vi "DriveLoop.vi"   [LabVIEW 2017]
uses:
  <userlib>/836-Library/System/QCP_V2/QCPSupportCode/QCP_GetDblArr.vi
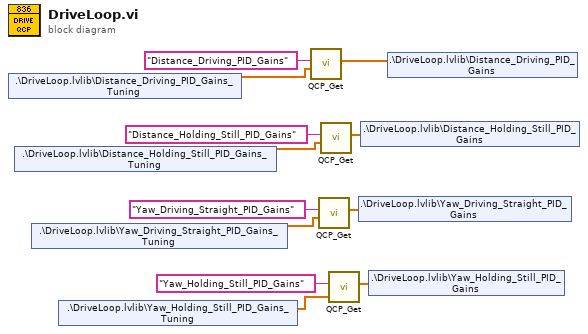
[diagram p0: block diagram]
diagram:
  n1 = shared-variable ".\\DriveLoop.lvlib\\Distance_Driving_PID_Gains_Tuning"() -> (w4:dbl[])  [unwired: 1 in, 1 out]
  n2 = shared-variable ".\\DriveLoop.lvlib\\Distance_Holding_Still_PID_Gains_Tuning"() -> (w3:dbl[])  [unwired: 1 in, 1 out]
  n3 = shared-variable ".\\DriveLoop.lvlib\\Yaw_Driving_Straight_PID_Gains_Tuning"() -> (w2:dbl[])  [unwired: 1 in, 1 out]
  n4 = shared-variable ".\\DriveLoop.lvlib\\Yaw_Holding_Still_PID_Gains_Tuning"() -> (w1:dbl[])  [unwired: 1 in, 1 out]
  n5 = call-poly <userlib>:"QCP_Get.vi"("Tuning Value"=w4, "Value Name"="Distance_Driving_PID_Gains") -> ("Values"=w8:dbl[])  [unwired: 7 in, 2 out]
  n6 = call-poly <userlib>:"QCP_Get.vi"("Tuning Value"=w2, "Value Name"="Yaw_Driving_Straight_PID_Gains") -> ("Values"=w6:dbl[])  [unwired: 7 in, 2 out]
  n7 = call-poly <userlib>:"QCP_Get.vi"("Tuning Value"=w3, "Value Name"="Distance_Holding_Still_PID_Gains") -> ("Values"=w7:dbl[])  [unwired: 7 in, 2 out]
  n8 = call-poly <userlib>:"QCP_Get.vi"("Tuning Value"=w1, "Value Name"="Yaw_Holding_Still_PID_Gains") -> ("Values"=w5:dbl[])  [unwired: 7 in, 2 out]
  n9 = shared-variable ".\\DriveLoop.lvlib\\Yaw_Driving_Straight_PID_Gains"(w6) -> ()  [unwired: 1 in, 1 out]
  n10 = shared-variable ".\\DriveLoop.lvlib\\Distance_Holding_Still_PID_Gains"(w7) -> ()  [unwired: 1 in, 1 out]
  n11 = shared-variable ".\\DriveLoop.lvlib\\Yaw_Holding_Still_PID_Gains"(w5) -> ()  [unwired: 1 in, 1 out]
  n12 = shared-variable ".\\DriveLoop.lvlib\\Distance_Driving_PID_Gains"(w8) -> ()  [unwired: 1 in, 1 out]
